vi "Read Motor Velocity.vi"(8 "error in (no error)":errorcluster, 10 "Motor ID (0)":u8, 11 "Dynamixel Motor Simulator in":refnum<class "Dynamixel Motor Simulator.lvclass">) -> (0 "error out":errorcluster, 2 "Velocity (RPM)":dbl, 3 "Dynamixel Motor Simulator out":refnum<class "Dynamixel Motor Simulator.lvclass">)   [LabVIEW 2016, in "Dynamixel Motor Simulator.lvclass"]
doc: "Retrieves the motor's velocity."
uses:
  <instrlib>/Dynamixel Motor/HAIOL/Simulator/Dynamixel Motor Simulator.lvclass
  <instrlib>/Dynamixel Motor/HAIOL/Simulator/Dynamixel Motor Simulator.lvclass/Dynamixel Motor Simulator.ctl
  <vilib>/robotics/Simulator/Robot Factory/Motor/ODESimulator_Motor.lvclass
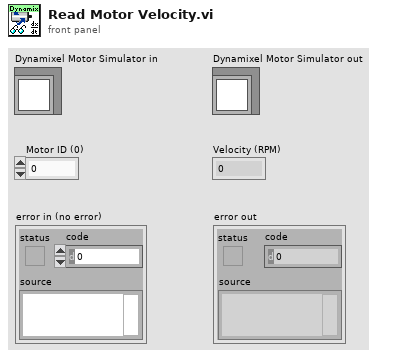
[diagram p1: front panel]
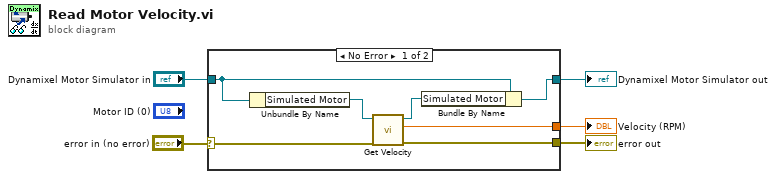
[diagram p0: block diagram]
diagram:
  n1 = case shown="No Error" "error in (no error)" {
    selector: "error in (no error)" -> [w12 w13]
    tunnel: "Dynamixel Motor Simulator in" -> [w8 w14]
    tunnel: [w11 w13] -> w3
    tunnel: [w7 w14] -> w2
    tunnel: [w6 _] -> w1
    frame No Error {
      n2 = Unbundle By Name(w8) -> ("Simulated Motor"=w10:refnum<class "ODESimulator_Motor.lvclass">)
      n3 = call-dynamic "Get Velocity.vi"("error in (no error)"=w12, "Motor in"=w10) -> ("error out"=w11:errorcluster, "CCW Velocity (rad/s)"=w6:dbl, "Motor out"=w9:refnum<class "ODESimulator_Motor.lvclass">)  [unwired: 7 in]
      n4 = Bundle By Name(cluster=w8, "Simulated Motor"=w9) -> (w7:refnum<class "Dynamixel Motor Simulator.lvclass">)
    }
    frame Error {
    }
  }
  "error out" <- w3
  "Dynamixel Motor Simulator out" <- w2
  "Velocity (RPM)" <- w1
